vi "To U16s.vi"(10 "Numeric":dbl, 11 "DataType":T1) -> (3 "Array":u16[](array[numeric]))   [LabVIEW 2020, in "Modbus Master Engine.lvlib"]
uses:
  Modbus Master Engine.lvlib
  Shared/Controls/Data Model/DataType.ctl
  Shared/Modbus Master Shared.lvlib
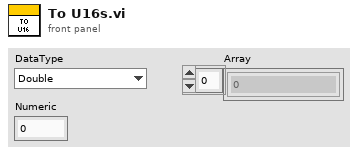
[diagram p1: front panel]
types:
  T1 = typedef "Modbus Master Shared.lvlib/DataType.ctl" = enum16{"Double", "Single", "I64", "I32", "I16", "I8", "U64", "U32", "U16", "U8", "Boolean"}
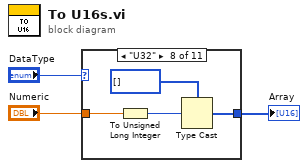
[diagram p0: block diagram]
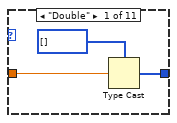
[diagram p2: hidden frame]
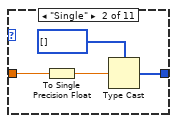
[diagram p3: hidden frame]
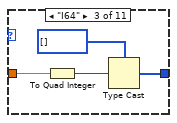
[diagram p4: hidden frame]
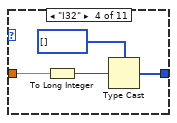
[diagram p5: hidden frame]
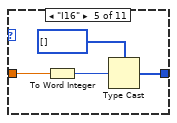
[diagram p6: hidden frame]
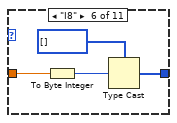
[diagram p7: hidden frame]
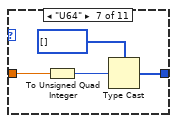
[diagram p8: hidden frame]
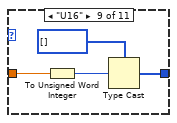
[diagram p9: hidden frame]
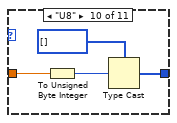
[diagram p10: hidden frame]
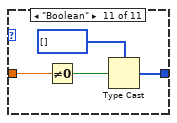
[diagram p11: hidden frame]
diagram:
  n1 = case shown="\"U32\"" "DataType" {
    tunnel: "Numeric" -> [w5 w8 w12 w16 w20 w24 w28 w32 w36 w40 w44]
    tunnel: [w4 w9 w13 w17 w21 w25 w29 w33 w37 w41 w45] -> w1
    frame "Double" {
      n2 = Type Cast(type=u16[] [] ("allocation"), x=w5) -> (*(type *) &x=w4:u16[])
    }
    frame "Single" {
      n3 = To Single Precision Float(number=w8) -> (single precision float=w7:sgl)
      n4 = Type Cast(type=u16[] [] ("allocation"), x=w7) -> (*(type *) &x=w9:u16[])
    }
    frame "I64" {
      n5 = To Quad Integer(1:w12) -> (0:w11:i64)
      n6 = Type Cast(type=u16[] [] ("allocation"), x=w11) -> (*(type *) &x=w13:u16[])
    }
    frame "I32" {
      n7 = To Long Integer(number=w16) -> (32bit integer=w15:i32)
      n8 = Type Cast(type=u16[] [] ("allocation"), x=w15) -> (*(type *) &x=w17:u16[])
    }
    frame "I16" {
      n9 = To Word Integer(number=w20) -> (16bit integer=w19:i16)
      n10 = Type Cast(type=u16[] [] ("allocation"), x=w19) -> (*(type *) &x=w21:u16[])
    }
    frame "I8" {
      n11 = To Byte Integer(number=w24) -> (8bit integer=w23:i8)
      n12 = Type Cast(type=u16[] [] ("allocation"), x=w23) -> (*(type *) &x=w25:u16[])
    }
    frame "U64" {
      n13 = To Unsigned Quad Integer(1:w28) -> (0:w27:u64)
      n14 = Type Cast(type=u16[] [] ("allocation"), x=w27) -> (*(type *) &x=w29:u16[])
    }
    frame "U32" {
      n15 = To Unsigned Long Integer(number=w32) -> (unsigned 32bit integer=w31:u32)
      n16 = Type Cast(type=u16[] [] ("allocation"), x=w31) -> (*(type *) &x=w33:u16[])
    }
    frame "U16" {
      n17 = To Unsigned Word Integer(number=w36) -> (unsigned 16bit integer=w35:u16)
      n18 = Type Cast(type=u16[] [] ("allocation"), x=w35) -> (*(type *) &x=w37:u16[])
    }
    frame "U8" {
      n19 = To Unsigned Byte Integer(number=w40) -> (unsigned 8bit integer=w39:u8)
      n20 = Type Cast(type=u16[] [] ("allocation"), x=w39) -> (*(type *) &x=w41:u16[])
    }
    frame "Boolean" {
      n21 = Not Equal To 0?(x=w44) -> (x != 0?=w43:bool)
      n22 = Type Cast(type=u16[] [] ("allocation"), x=w43) -> (*(type *) &x=w45:u16[])
    }
  }
  "Array" <- w1
